vi "Test Worker Job Count Incremented.vi"(8 "error in (no error)":errorcluster, 11 "Worker Test in":refnum<class "Worker Test.lvclass">) -> (0 "error out":errorcluster, 3 "Worker Test out":refnum<class "Worker Test.lvclass">)   [LabVIEW 2020, in "Worker Test.lvclass"]
uses:
  Worker Test.lvclass
  <vilib>/Asteme/Triarc Framework/Process/Process.lvclass
  Worker/Worker.lvclass
  <vilib>/Asteme/Triarc Framework Test Suite/Support/Event Helpers/Event Helpers.lvlib
  C:/Users/anton/Documents/GitHub/Triarc-Examples/Coffee Shop/Person/Person.lvclass
  C:/Program Files (x86)/National Instruments/LabVIEW 2020/vi.lib/Asteme/Triarc Framework/View/View.lvclass
  C:/Program Files (x86)/National Instruments/LabVIEW 2020/vi.lib/Asteme/Triarc Framework/Process/Process.lvclass
  C:/Program Files (x86)/National Instruments/LabVIEW 2020/vi.lib/Asteme/Triarc Framework/Base/Base.lvclass
  C:/Program Files (x86)/National Instruments/LabVIEW 2020/vi.lib/Asteme/Triarc Framework/Error Handler Interface/Error Handler Interface.lvclass
  C:/Program Files (x86)/National Instruments/LabVIEW 2020/vi.lib/Asteme/Triarc Framework/Logging/Logging.lvclass
  C:/Users/anton/Documents/GitHub/Triarc-Examples/Coffee Shop/Worker/Worker.lvclass
  <vilib>/Asteme/LUnit/Test Case.lvclass
  C:/Users/anton/Documents/GitHub/Triarc-Examples/Coffee Shop/Person Test/Person Test.lvclass
  C:/Program Files (x86)/National Instruments/LabVIEW 2020/vi.lib/Asteme/Triarc Framework Test Suite/View Test/View Test.lvclass
  C:/Program Files (x86)/National Instruments/LabVIEW 2020/vi.lib/Asteme/Triarc Framework Test Suite/Process Test/Process Test.lvclass
  C:/Program Files (x86)/National Instruments/LabVIEW 2020/vi.lib/Asteme/Triarc Framework Test Suite/Base Class Test/Base Test.lvclass
  C:/Program Files (x86)/National Instruments/LabVIEW 2020/vi.lib/Asteme/LUnit/Test Case.lvclass
  C:/Users/anton/Documents/GitHub/Triarc-Examples/Coffee Shop/Worker Test/Worker Test.lvclass
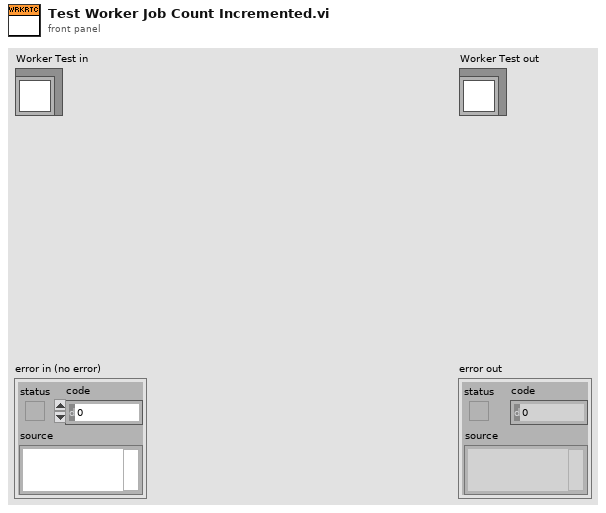
[diagram p1: front panel]
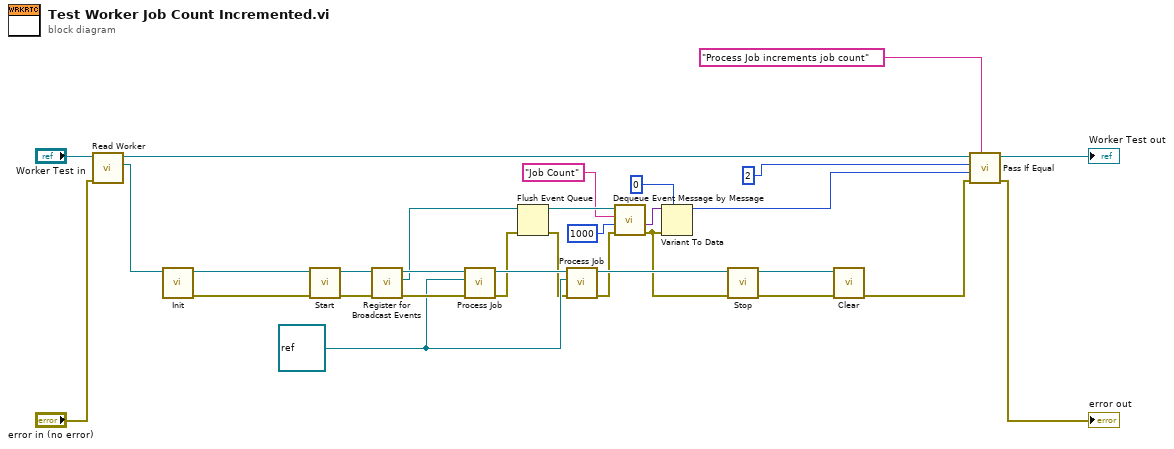
[diagram p0: block diagram]
diagram:
  w12 = refnum<class> refnum ("Task")
  n1 = call "Read Worker.vi"("error in (no error)"="error in (no error)", "Worker Test in"="Worker Test in") -> ("Worker"=w19:refnum<class "Worker.lvclass">, "Worker Test out"=w22:refnum<class "Worker Test.lvclass">)  [unwired: 7 in, 1 out]
  n2 = call-dynamic "Init.vi"("View In"=w19) -> ("error out"=w31:errorcluster, "View Out"=w26:refnum<class "Worker.lvclass">)  [unwired: 9 in]
  n3 = call <vilib>:"Start.vi"("error in (no error)"=w31, "Process In"=w26) -> ("error out"=w25:errorcluster, "Process Out"=w17:refnum<class "Worker.lvclass">)  [unwired: 8 in]
  n4 = call <vilib>:"Register for Broadcast Events.vi"("error in (no error)"=w25, "Process In"=w17) -> ("error out"=w18:errorcluster, "Event Registration Refnum Out"=w10:refnum<event-registration>, "Process Out"=w16:refnum<class "Worker.lvclass">)  [unwired: 7 in]
  n5 = call "Process Job.vi"("error in (no error)"=w18, "Task"=w12, "Worker In"=w16) -> ("error out"=w14:errorcluster, "Worker Out"=w15:refnum<class "Worker.lvclass">)  [unwired: 7 in]
  n6 = Flush Event Queue(0:w10, 3:w14) -> (8:w9:refnum<event-registration>, 11:w11:errorcluster)  [unwired: 4 in, 1 out]
  n7 = call "Process Job.vi"("error in (no error)"=w11, "Task"=w12, "Worker In"=w15) -> ("error out"=w6:errorcluster, "Worker Out"=w13:refnum<class "Worker.lvclass">)  [unwired: 7 in]
  n8 = call <vilib>:"Dequeue Event Message by Message.vi"("error in (no error)"=w6, "Timeout (-1)"=1000, "Message"="Job Count", "Event Registration Refnum"=w9) -> ("error out"=w1:errorcluster, "Message Data"=w5:variant)  [unwired: 3 in, 3 out]
  n9 = Variant To Data(error in=w1, type=u32 0 ("code"), Variant=w5) -> (data=w3:u32)  [unwired: 1 out]
  n10 = call <vilib>:"Stop.vi"("error in (no error)"=w1, "Process In"=w13) -> ("error out"=w29:errorcluster, "Process Out"=w30:refnum<class "Worker.lvclass">)  [unwired: 7 in, 1 out]
  n11 = call-dynamic "Clear.vi"("error in (no error)"=w29, "View In"=w30) -> ("error out"=w24:errorcluster)  [unwired: 9 in]
  n12 = call <vilib>:"Pass If Equal.vi"("Description"="Process Job increments job count", "error in (no error)"=w24, "Actual"=w3, "Expected"=u32 2 ("code"), "Test Case In"=w22) -> ("error out"=→"error out":errorcluster, "Test Case Out"=→"Worker Test out":refnum<class "Worker Test.lvclass">)  [unwired: 5 in]
